vi "OE 3 (2).vi"() -> ()   [LabVIEW 2021]
panel:
  in  "Frequency":dbl
  out "Waveform Graph":dbl[](graph)
  in  "Amplitude":dbl
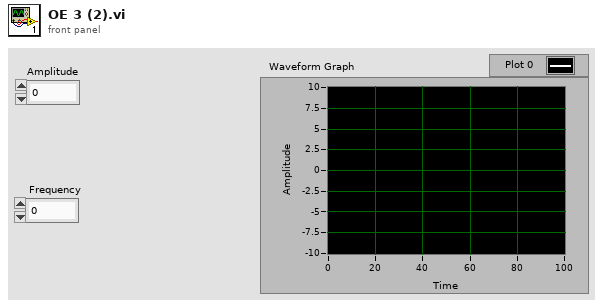
[diagram p1: front panel]
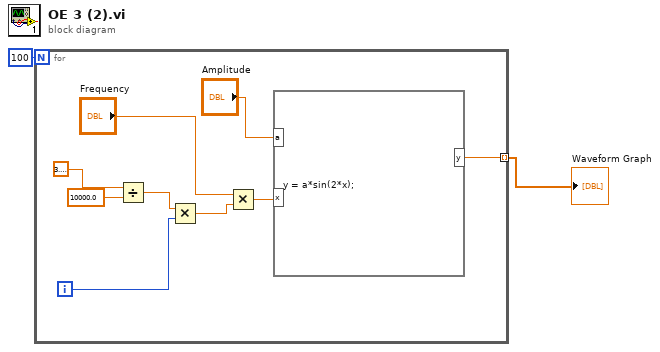
[diagram p0: block diagram]
diagram:
  n1 = for {
    N: 100 -> [_]
    tunnel: [w11] -> w2 mode=indexing
    i -> [w8]
    n2 = Divide(x=3.141592653589793, y=10000.0) -> (x/y=w7:dbl)
    n3 = Multiply(x=w7, y=w8) -> (x*y=w5:dbl)
    n4 = Multiply(x="Frequency", y=w5) -> (x*y=w6:dbl)
    n5 = formula code="y = a*sin(2*x);"("x"=w6, "a"="Amplitude") -> ("y"=w11:dbl)
  }
  "Waveform Graph" <- w2
